vi "Write Ready for iterations.vi"(8 "error in (no error)":errorcluster, 10 "Ready for iterations":bool, 11 "Example Actor in":refnum<class "Example Actor.lvclass">) -> (0 "error out":errorcluster, 3 "Example Actor out":refnum<class "Example Actor.lvclass">)   [LabVIEW 2021, in "Example Iterator NR Actor Explicit Iteration.lvlib" / "Example Actor.lvclass"]
uses:
  Example Actor.lvclass
  Example Actor.lvclass/Example Actor.ctl
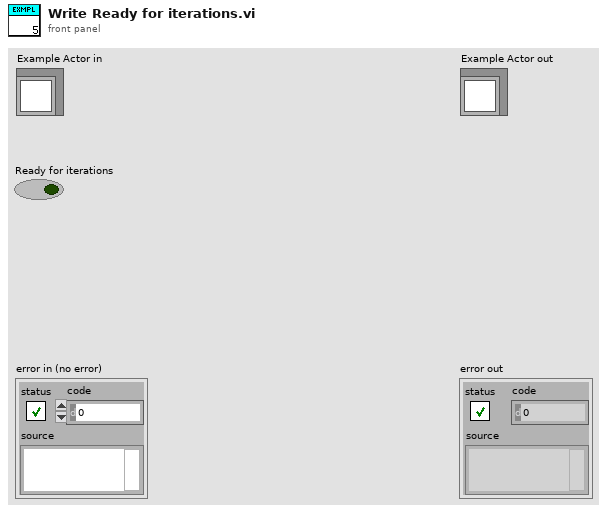
[diagram p1: front panel]
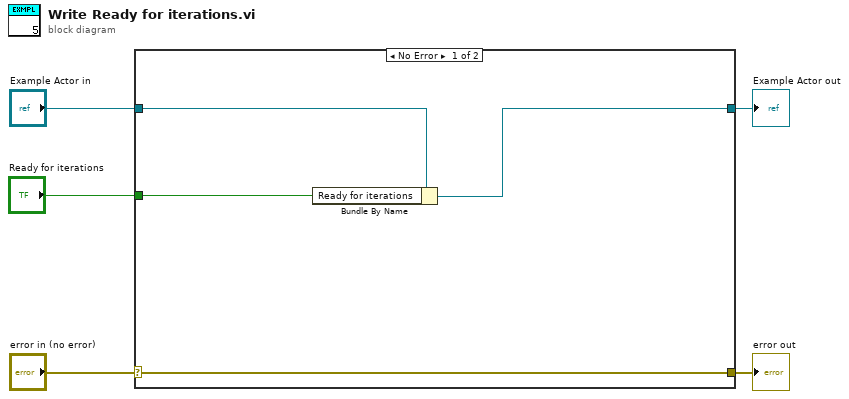
[diagram p0: block diagram]
diagram:
  n1 = case shown="No Error" "error in (no error)" {
    selector: "error in (no error)" -> [w9 w11]
    tunnel: [w9 w11] -> w4
    tunnel: [w7 w10] -> w2
    tunnel: "Example Actor in" -> [w8 w10]
    tunnel: "Ready for iterations" -> [w6 _]
    frame No Error {
      n2 = Bundle By Name(cluster=w8, "Ready for iterations"=w6) -> (w7:refnum<class "Example Actor.lvclass">)
    }
    frame Error {
    }
  }
  "error out" <- w4
  "Example Actor out" <- w2
